vi "Calculate z coord_v2.vi"(4 "Z factor":dbl[](array[numeric]), 6 "Z coord info":dbl[](array[numeric]), 7 "current (x,y)":dbl[](array[numeric]), 8 "xy grid min":dbl[](array[numeric]), 9 "index factor (DBL)":dbl, 10 "Za array":dbl[][](array[numeric]), 11 "Zp array":dbl[][](array[numeric])) -> (1 "za":dbl, 2 "zp":dbl, 3 "cal z":dbl)   [LabVIEW 2010]
doc: "This VI computes the adaptive z coordinate value based on current (x,y) coordinate.\nv2 version is used for scooping motion.\n\"Z coord info\" = [zp_eps, za_eps,zi]\nzp_eps: bound to posterior capsule\nza_eps: bound to anterior capsule\nzi: starting z coordinate of the trajectory"
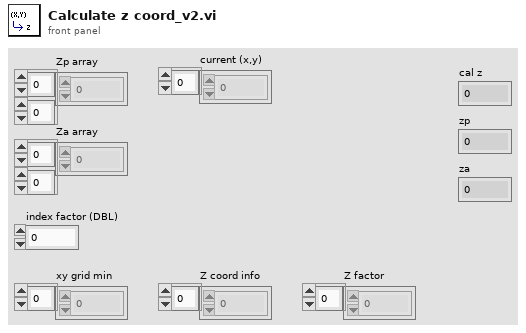
[diagram p1: front panel]
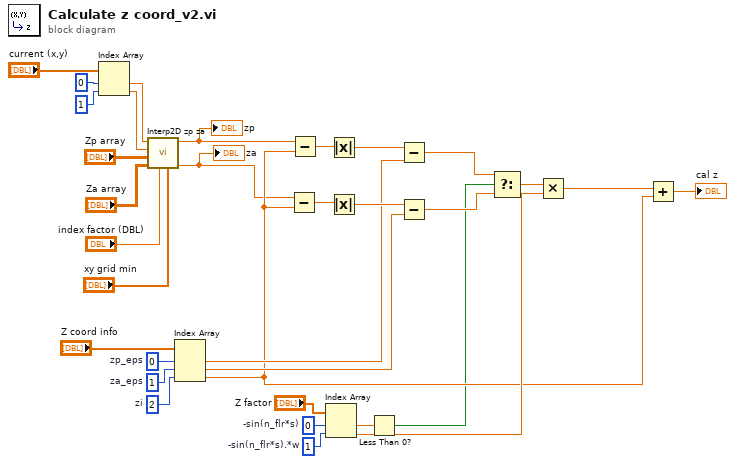
[diagram p0: block diagram]
diagram:
  w20 = 1  # -sin(n_flr*s).*w
  w19 = 0  # -sin(n_flr*s)
  w23 = 2  # zi
  w24 = 1  # za_eps
  w25 = 0  # zp_eps
  n1 = Index Array(array="current (x,y)", index #1=0 ("index"), index #2=1 ("index")) -> (element #1=w28:dbl, element #2=w27:dbl)
  n2 = call "Interp2D zp za.vi"("xy grid min"="xy grid min", "index factor (DBL)"="index factor (DBL)", "Za array"="Za array", "Zp array"="Zp array", "current y"=w27, "current x"=w28) -> ("za"=w2:dbl, "zp"=w3:dbl)  [unwired: 4 in]
  "zp" <- w3
  "za" <- w2
  n3 = Index Array(array="Z coord info", index #1=w25, index #2=w24, index #3=w23) -> (element #1=w13:dbl, element #2=w12:dbl, element #3=w7:dbl)
  n4 = Subtract(x=w2, y=w7) -> (x-y=w16:dbl)
  n5 = Subtract(x=w3, y=w7) -> (x-y=w17:dbl)
  n6 = Index Array(array="Z factor", index #1=w19, index #2=w20) -> (element #1=w4:dbl, element #2=w9:dbl)
  n7 = Absolute Value(x=w17) -> (abs(x)=w15:dbl)
  n8 = Absolute Value(x=w16) -> (abs(x)=w14:dbl)
  n9 = Less Than 0?(x=w4) -> (x < 0?=w5:bool)
  n10 = Subtract(x=w15, y=w13) -> (x-y=w11:dbl)
  n11 = Subtract(x=w14, y=w12) -> (x-y=w10:dbl)
  n12 = Select(t=w11, s=w5, f=w10) -> (s? t:f=w8:dbl)
  n13 = Multiply(x=w8, y=w9) -> (x*y=w1:dbl)
  n14 = Add(x=w1, y=w7) -> (x+y=→"cal z":dbl)
